vi "niDTS BT INSTR TX Configure IBE.vi"(8 "error in (no error)":errorcluster, 11 "niDTS BT INSTR TX in":refnum<class "niDTS BT INSTR TX.lvclass">) -> (0 "error out":errorcluster, 3 "niDTS BT INSTR TX out":refnum<class "niDTS BT INSTR TX.lvclass">)   [LabVIEW 2015, in "niDTS BT.lvlib" / "niDTS BT INSTR TX.lvclass"]
doc: "Sets:\n\n* TriggerThreshold\n* Trigger Source\n* MinQuietTimeDuration\n* TriggerTimeout"
uses:
  niDTS BT INSTR TX.lvclass
  niDTS BT INSTR TX.lvclass/niDTS BT INSTR TX.ctl
  RiviInstDriver/niRfsaBT/Objects/niRfsaBt.lvclass
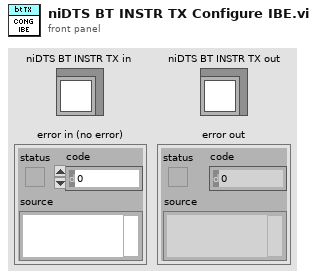
[diagram p1: front panel]
types:
  T1 = typedef "niRfsaBT.lvclass/niRfsaBT INC Handle.ctl" = refnum<data-value>
  T2 = enum16{"RMS", "LOG", "SCALAR", "MAX", "MIN", "VECTOR"}
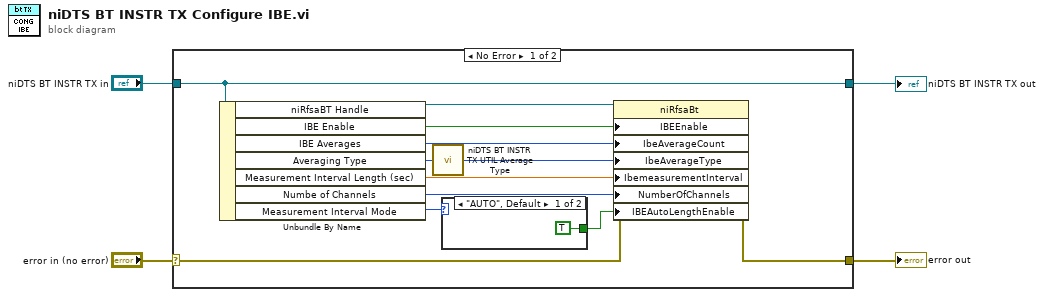
[diagram p0: block diagram]
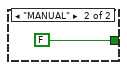
[diagram p2: hidden frame]
diagram:
  n1 = case shown="No Error" "error in (no error)" {
    selector: "error in (no error)" -> [w16 w20]
    tunnel: [w15 w20] -> w3
    tunnel: "niDTS BT INSTR TX in" -> [w13 w19]
    tunnel: [w13 w19] -> w1
    frame No Error {
      n2 = Unbundle By Name(w13) -> ("niRfsaBT Handle"=w14:T1, "IBE Enable"=w12:bool, "IBE Averages"=w10:i32, "Averaging Type"=w11:T2, "Measurement Interval Length (sec)"=w8:dbl, "Numbe of Channels"=w7:i32, "Measurement Interval Mode"=w6:enum16{"AUTO", "MANUAL"})
      n3 = call "niDTS BT INSTR TX UTIL Average Type.vi"("Type In"=w11) -> ("Type Out"=w9:enum16{"RMS", "LOG", "SCALar", "MAX", "MIN"})  [unwired: 14 in]
      n4 = case shown="\"AUTO\", Default" w6 {
        tunnel: [TRUE ("CONFigure:RFSA:BLUetooth:MEASurement:IBEMissions:INTerval:LENGth:AUTO:IBEAutoLengthEnable") FALSE ("CONFigure:RFSA:BLUetooth:MEASurement:IBEMissions:INTerval:LENGth:AUTO:IBEAutoLengthEnable")] -> w5
        frame "AUTO", Default {
        }
        frame "MANUAL" {
        }
      }
      n5 = property class="niRfsaBt"(reference=w14, error in=w16, "IBEEnable"=w12, "IbeAverageCount"=w10, "IbeAverageType"=w9, "IbemeasurementInterval"=w8, "NumberOfChannels"=w7, "IBEAutoLengthEnable"=w5) -> (error out=w15:errorcluster)  [unwired: 1 out]
    }
    frame Error {
    }
  }
  "error out" <- w3
  "niDTS BT INSTR TX out" <- w1
